vi "Encode CONT Parameters.vi"(6 "Internal Scanner Exists?":bool=TRUE, 8 "ADD Parameters (in)":string, 10 "Scanner Settings":T2={"Scan1"=1, "Scan2"=1, "Scan3"=1, "Scan4"=1, "Scan5"=1, "Scan6"=1, "Scan7"=1, "Scan8"=1, "Scan9"=1, "Scan10"=1, "Scan11"=1, "Scan12"=1, "Scan13"=1, "Scan14"=1, "Scan15"=1, "Scan16"=1} {"Scan16" scale=0.0..2.0; "Scan15" scale=0.0..2.0; "Scan14" scale=0.0..2.0; "Scan13" scale=0.0..2.0; "Scan12" scale=0.0..2.0; "Scan11" scale=0.0..2.0; "Scan10" scale=0.0..2.0; "Scan9" scale=0.0..2.0; "Scan8" scale=0.0..2.0; "Scan7" scale=0.0..2.0; "Scan6" scale=0.0..2.0; "Scan5" scale=0.0..2.0; "Scan4" scale=0.0..2.0; "Scan3" min=0 max=2 scale=0.0..2.0; "Scan2" min=0 max=2 scale=0.0..2.0; "Scan1" min=0 max=2 scale=0.0..2.0}, 11 "Continuity Test Paramameters in":T1={"High Limit (0 - 10,000 ohms) (1000)"=1000.0, "Low Limit (0 - 10,000 ohms) (0)"=0.0, "Dwell Time (0.0, 0.4 - 999.9 seconds) (1.0)"=1.0, "Offset (0 - 10.00 ohms) (0)"=0.0, "Auto Offset (F: Off)"=FALSE} {"Offset (0 - 10.00 ohms) (0)" format="%.2f"; "Dwell Time (0.0, 0.4 - 999.9 seconds) (1.0)" format="%.1f"; "Low Limit (0 - 10,000 ohms) (0)" format="%.2f"; "High Limit (0 - 10,000 ohms) (1000)" format="%.2f"}) -> (0 "Scanner Settings out":T2={"Scan1"=1, "Scan2"=1, "Scan3"=1, "Scan4"=1, "Scan5"=1, "Scan6"=1, "Scan7"=1, "Scan8"=1, "Scan9"=1, "Scan10"=1, "Scan11"=1, "Scan12"=1, "Scan13"=1, "Scan14"=1, "Scan15"=1, "Scan16"=1} {"Scan16" scale=0.0..2.0; "Scan15" scale=0.0..2.0; "Scan14" scale=0.0..2.0; "Scan13" scale=0.0..2.0; "Scan12" scale=0.0..2.0; "Scan11" scale=0.0..2.0; "Scan10" scale=0.0..2.0; "Scan9" scale=0.0..2.0; "Scan8" scale=0.0..2.0; "Scan7" scale=0.0..2.0; "Scan6" scale=0.0..2.0; "Scan5" scale=0.0..2.0; "Scan4" scale=0.0..2.0; "Scan3" min=0 max=2 scale=0.0..2.0; "Scan2" min=0 max=2 scale=0.0..2.0; "Scan1" min=0 max=2 scale=0.0..2.0}, 1 "Continuity Test Paramameters out":T1={"High Limit (0 - 10,000 ohms) (1000)"=1000.0, "Low Limit (0 - 10,000 ohms) (0)"=0.0, "Dwell Time (0.0, 0.4 - 999.9 seconds) (1.0)"=1.0, "Offset (0 - 10.00 ohms) (0)"=0.0, "Auto Offset (F: Off)"=FALSE} {"Offset (0 - 10.00 ohms) (0)" format="%.2f"; "Dwell Time (0.0, 0.4 - 999.9 seconds) (1.0)" format="%.1f"; "Low Limit (0 - 10,000 ohms) (0)" format="%.2f"; "High Limit (0 - 10,000 ohms) (1000)" format="%.2f"}, 3 "Add Step":string)   [LabVIEW 2012, in "Associated Research 78XX Series.lvlib"]
uses:
  <instrlib>/Associated Research 78XX Series/Associated Research 78XX Series.lvlib
  <instrlib>/Associated Research 78XX Series/Public/Configure/Steps/Low Level/Scanner Settings.ctl
  <instrlib>/Associated Research 78XX Series/Public/Configure/Steps/Low Level/CONT Test Parameters.ctl
panel:
  # "On\nOff"
  # "On\nOff"
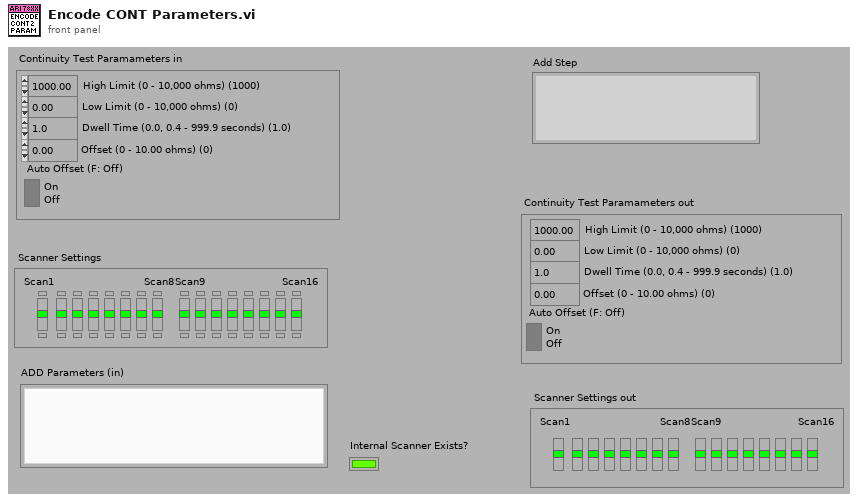
[diagram p1: front panel]
types:
  T1 = typedef "Associated Research 78XX Series.lvlib/CONT Test Parameters.ctl" = cluster{"High Limit (0 - 10,000 ohms) (1000)":dbl, "Low Limit (0 - 10,000 ohms) (0)":dbl, "Dwell Time (0.0, 0.4 - 999.9 seconds) (1.0)":dbl, "Offset (0 - 10.00 ohms) (0)":dbl, "Auto Offset (F: Off)":bool}
  T2 = typedef "Associated Research 78XX Series.lvlib/Scanner Settings.ctl" = cluster{"Scan1":i32, "Scan2":i32, "Scan3":i32, "Scan4":i32, "Scan5":i32, "Scan6":i32, "Scan7":i32, "Scan8":i32, "Scan9":i32, "Scan10":i32, "Scan11":i32, "Scan12":i32, "Scan13":i32, "Scan14":i32, "Scan15":i32, "Scan16":i32}
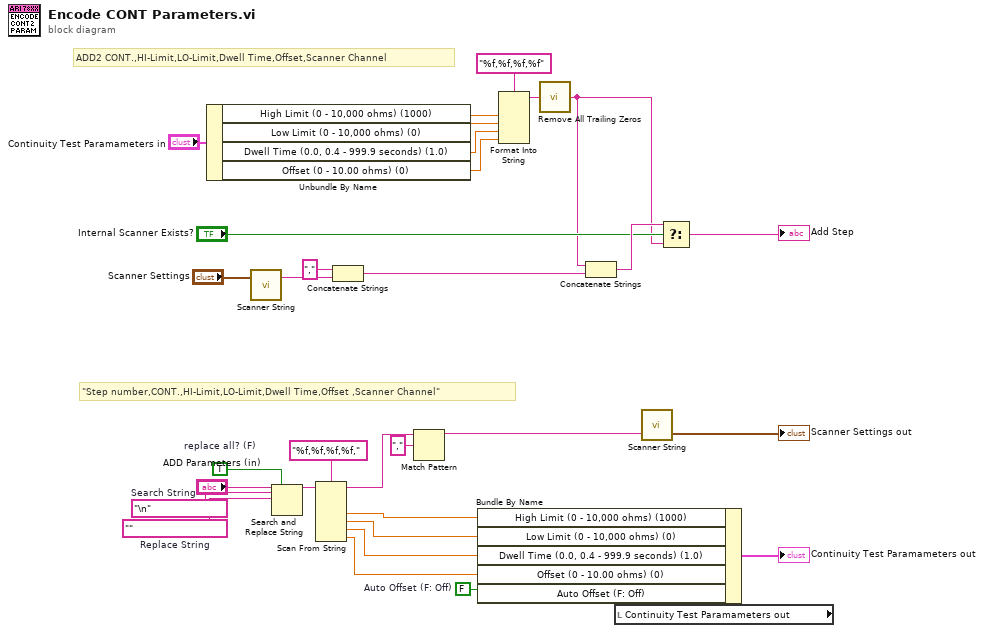
[diagram p0: block diagram]
diagram:
  w17 = TRUE  # replace all? (F)
  w18 = ""  # Replace String
  w19 = "\n"  # Search String
  w20 = FALSE  # Auto Offset (F: Off)
  # "\"Step number,CONT.,HI-Limit,LO-Limit,Dwell Time,Offset ,Scanner Channel\""
  # "ADD2 CONT.,HI-Limit,LO-Limit,Dwell Time,Offset,Scanner Channel"
  n1 = Unbundle By Name("Continuity Test Paramameters in") -> ("High Limit (0 - 10,000 ohms) (1000)"=w32:dbl, "Low Limit (0 - 10,000 ohms) (0)"=w31:dbl, "Dwell Time (0.0, 0.4 - 999.9 seconds) (1.0)"=w30:dbl, "Offset (0 - 10.00 ohms) (0)"=w29:dbl)
  n2 = call <instrlib>:"Scanner String.vi"("Scanner Settings in"="Scanner Settings") -> ("Scanner String (out)"=w10:string)  [unwired: 1 in, 1 out]
  n3 = Search and Replace String(replace all?=w17, input string="ADD Parameters (in)", search string=w19, replace string=w18) -> (result string=w15:string)  [unwired: 4 in, 3 out]
  n4 = Scan From String(format string="%f,%f,%f,%f," ("Format String"), input string=w15) -> (remaining string=w12:string, output 1=w24:dbl, output 2=w23:dbl, output 3=w22:dbl, output 4=w21:dbl)  [unwired: 6 in, 2 out]
  n5 = Concatenate Strings("," ("string"), w10) -> (w7:string)
  n6 = Match Pattern(string=w12, regular expression=",") -> (before substring=w6:string)  [unwired: 1 in, 3 out]
  n7 = Format Into String(format string="%f,%f,%f,%f" ("Format String"), w32, w31, w30, w29) -> (resulting string=w27:string)  [unwired: 2 in, 1 out]
  n8 = call <instrlib>:"Remove All Trailing Zeros.vi"("String in"=w27) -> ("String out"=w8:string)
  n9 = Concatenate Strings(w8, w7) -> (w26:string)
  n10 = local read "Continuity Test Paramameters out"() -> (w14:T1)
  n11 = Bundle By Name(cluster=w14, "High Limit (0 - 10,000 ohms) (1000)"=w24, "Low Limit (0 - 10,000 ohms) (0)"=w23, "Dwell Time (0.0, 0.4 - 999.9 seconds) (1.0)"=w22, "Offset (0 - 10.00 ohms) (0)"=w21, "Auto Offset (F: Off)"=w20) -> (→"Continuity Test Paramameters out":T1)
  n12 = call <instrlib>:"Scanner String.vi"("Scanner String (in)"=w6) -> ("Scanner Settings out"=→"Scanner Settings out":T2)  [unwired: 1 in, 1 out]
  n13 = Select(t=w26, s="Internal Scanner Exists?", f=w8) -> (s? t:f=→"Add Step":string)
